vi "OAT Adjust Position and Range.vi"(7 "reset":bool, 9 "range in":cluster{"start":dbl, "end":dbl, "step":dbl} {"step" format="%.2f"; "end" format="%.2f"; "start" format="%.2f"}, 10 "start position":dbl format="%.2f", 11 "current position":dbl format="%.2f") -> (0 "flags":cluster{"finished":bool, "data missed":bool}, 1 "range out":cluster{"start":dbl, "end":dbl, "step":dbl} {"step" format="%.2f"; "end" format="%.2f"; "start" format="%.2f"}, 2 "scale":cluster{"offset":dbl, "multiplier":dbl} {"multiplier" format="%.2f"; "offset" format="%.2f"}, 3 "current position out":dbl format="%.2f")   [LabVIEW 2017]
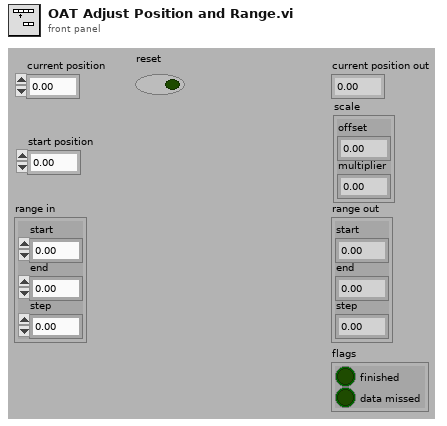
[diagram p1: front panel]
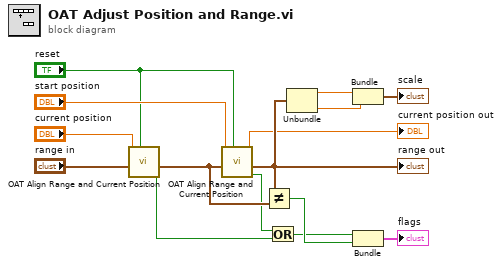
[diagram p0: block diagram]
diagram:
  n1 = call <vilib>:"OAT Align Range and Current Position.vi"("reset"="reset", "range"="range in", "current position"="current position") -> ("range empty?"=w3:bool, "new range"=w5:cluster{"start":dbl, "end":dbl, "step":dbl})  [unwired: 6 in, 1 out]
  n2 = call <vilib>:"OAT Align Range and Current Position.vi"("reset"="reset", "range"=w5, "current position"="start position") -> ("range empty?"=w4:bool, "new range"=w14:cluster{"start":dbl, "end":dbl, "step":dbl}, "position out"=→"current position out":dbl)  [unwired: 6 in]
  "range out" <- w14
  n3 = Not Equal?(x=w14, y=w5) -> (x != y?=w10:bool)
  n4 = Or(x=w4, y=w3) -> (x .or. y?=w2:bool)
  n5 = Unbundle(w14) -> ("start"=w13:dbl, "step"=w12:dbl)  [unwired: 1 out]
  n6 = Bundle("start"=w13, "step"=w12) -> (→"scale":cluster{"start":dbl, "step":dbl})  [unwired: 1 in]
  n7 = Bundle(w2, w10) -> (→"flags":cluster{bool, bool})  [unwired: 1 in]
